vi "ZZZ Chroma 1905x Series Status-.vi"(3 "error in":T1, 5 "inst handle in":refnum<visa-resource-name>) -> (0 "error out":T1, 1 "Status":string, 2 "inst handle out":refnum<visa-resource-name>)   [LabVIEW 2025]
panel:
  # "Status?"
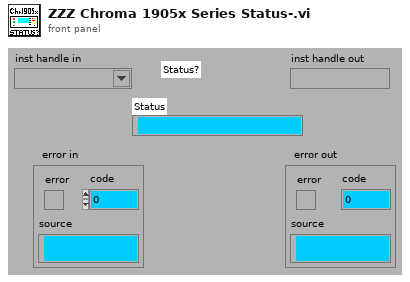
[diagram p1: front panel]
types:
  T1 = cluster{"error":bool, "code":i8, "source":string}
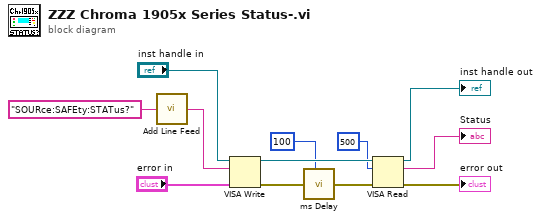
[diagram p0: block diagram]
diagram:
  n1 = call <instrlib>:"Add Line Feed.vi"("Command string"="SOURce:SAFEty:STATus?") -> ("Concatenated string"=w5:string)  [unwired: 4 in]
  n2 = VISA Write(VISA resource name="inst handle in", write buffer=w5, error in (no error)="error in") -> (VISA resource name out=w12:refnum<visa-resource-name>, error out=w3:errorcluster)  [unwired: 1 out]
  n3 = call <instrlib>:"ms Delay.vi"("miliseconds to wait"=u32 100, "error in (no error)"=w3) -> ("error out"=w2:errorcluster)  [unwired: 6 in, 1 out]
  n4 = VISA Read(VISA resource name=w12, byte count=u32 500 ("byte count (0)"), error in (no error)=w2) -> (VISA resource name out=→"inst handle out":refnum<visa-resource-name>, read buffer=→"Status":string, error out=→"error out":errorcluster)  [unwired: 1 out]
